vi "Read (I16 Data Ref).vi"(0 "disk streaming in":refnum<class "Disk Streaming.lvclass">, 1 "sample data":refnum<data-value>, 2 "elements in region":u32, 3 "empty elements remaining":u32, 5 "error in (no error)":errorcluster) -> (13 "finished":bool, 14 "disk streaming out":refnum<class "Disk Streaming.lvclass">, 18 "number of pending reads":u32, 19 "error out":errorcluster)   [LabVIEW 2021, in "Disk Streaming.lvclass"]
doc: "Reads data from a file in the streaming process controlled by a disk streaming instance and generates status information. For more information about the disk streaming instance refer to the <B>Open.vi</B> context help.\n\nUse this VI when streaming from disk using the TDMS Advanced Data Reference I/O functions (the disk streaming instance was created by the <B>Open.vi</B> with the <B>disk read (F) / write (T)</B> input set to false and the <B>I/O mode</B> input set to \"Data Reference\"). The streaming process requires the execution of the following sequence in a loop:\n1. Use the <B>Get Next Transfer Size.vi</B> to obtain the number of elements to transfer in the current iteration. If this VI returns zero, then the streaming is complete.\n2. Call the Acquire Write Region FIFO method on the Host to Target FIFO transferring the data to the FPGA Target to acquire the buffer to write with the data read from the file. Use the value returned by the <B>Get Next Transfer Size.vi</B> on the \"Number of Elements\" input of the FIFO method.\n3. Call this VI using the outputs returned by the FIFO method.\n\nInputs:\n\n<B>disk streaming in</B>: Disk streaming instance input.\n\n<B>sample data</B>: External Data Value Reference (EDVR) referencing the array of I16s to write with the data read from the file. Wire the \"Write Region Reference\" output of the FIFO method acquiring the Host to Target FIFO buffer to write to this input.\n\n<B>elements in region</B>: The size of the array of I16s referenced by the EDVR passed on the <B>sample data</B> input. Wire the \"Elements In Region\" output of the FIFO method acquiring the Host to Target FIFO buffer to write to this input.\n\n<B>empty elements remaining</B>: Set this input to the number of additional empty elements remaining in the host DMA buffer that are available for writing. This input is used only in the calculation of the Host DMA buffer utilization status. Wire the \"Empty Elements Remaining\" output of the FIFO method acquiring the Host to Target FIFO buffer to write to this input.\n\nOutputs:\n\n<B>disk streaming out</B>: Disk streaming instance output. Pass this output to the other Disk Streaming VIs to perform the streaming.\n\n<B>number of pending reads</B>: The number of asynchronous reads that are currently running in the background. Use the <B>Get Status.vi</B> to obtain additional status information.\n\n<B>finished</B>: Indicates whether the streaming is finished."
uses:
  Disk Streaming.lvclass
  Disk Streaming.lvclass/Disk Streaming.ctl
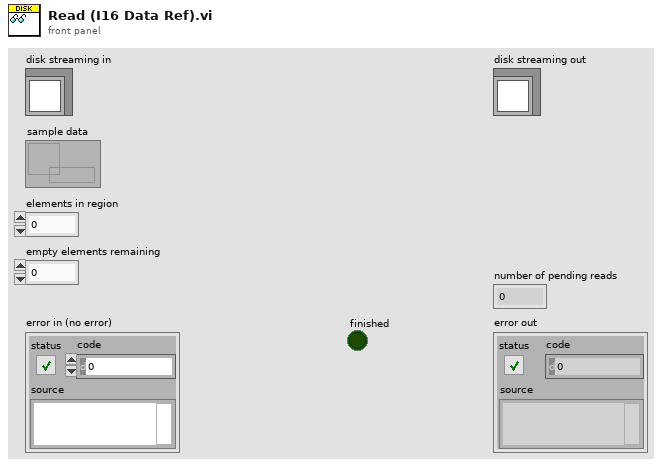
[diagram p1: front panel]
types:
  T1 = typedef "Disk Streaming.lvclass/Data.ctl" = cluster{"tdms file":refnum<k34>, "group name":string, "channel name":string, "max operations":u32, "timeout (s)":dbl, "data type size (bytes)":u64, "writing":bool, "I/O mode":T2, "# of blocks":u32, "block size divisor (bytes)":u32, "file position (elements)":u64, "file size (elements)":i64, "file size (samples)":i64, "block size (elements)":u64, "block size (samples)":u64, "quantum size (elements)":u64, "quantum size (samples)":u64, "samples remaining":i64, "elements transferred":u64, "finished":bool, "preview size":i32, "preview quantum size (elements)":u64, "preview quantum size (samples)":u64, "DMA buffer size (elements)":u32, "pending block sizes (bytes)":u64[]}
  T2 = typedef "Disk Streaming.lvclass/IO mode.ctl" = enum16{"Synchronous", "Asynchronous", "Data Reference"}
  T3 = typedef "Disk Streaming.lvclass/Status.ctl" = cluster{"finished":bool, "Host DMA buffer size (bytes)":u64, "Host DMA buffer utilization (bytes)":u64, "Disk maximum async operations":u32, "Disk pending async operations":u32, "preview data":i16[]}
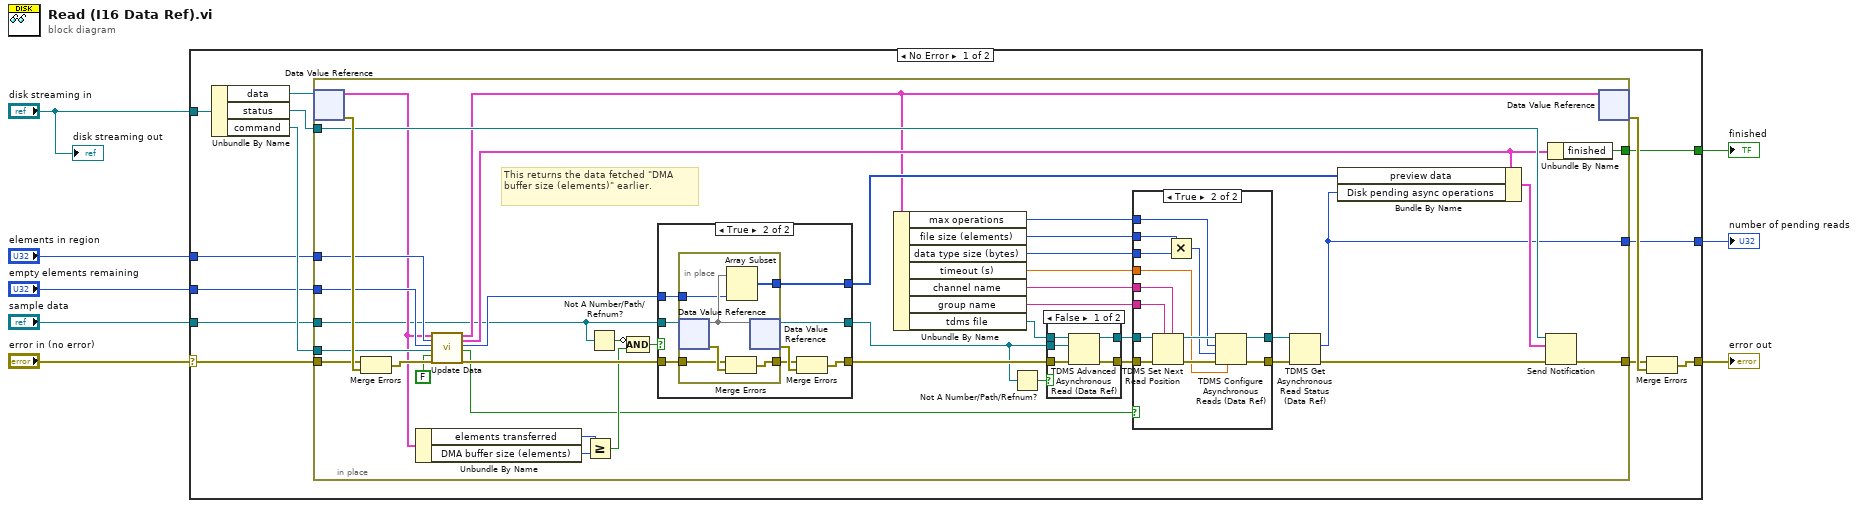
[diagram p0: block diagram]
diagram:
  n1 = case shown="No Error" "error in (no error)" {
    selector: "error in (no error)" -> [w19 w100]
    tunnel: [w18 w100] -> w7
    tunnel: [w16 _] -> w6
    tunnel: "empty elements remaining" -> [w13 _]
    tunnel: "disk streaming in" -> [w15 _]
    tunnel: [w11 _] -> w3
    tunnel: "sample data" -> [w10 _]
    tunnel: "elements in region" -> [w9 _]
    frame No Error {
      n2 = Unbundle By Name(w15) -> ("data"=w14:refnum<data-value>, "status"=w12:refnum<notifier>, "command"=w21:refnum<notifier>)
      n3 = in-place {
        in-place-border: w19 -> [w56]
        in-place-border: [w51] -> w17
        in-place-border: [w35] -> w16
        in-place-border: w21 -> [w53]
        in-place-border: w13 -> [w54]
        in-place-border: w12 -> [w57]
        in-place-border: [w50] -> w11
        in-place-border: w10 -> [w25]
        in-place-border: w9 -> [w44]
        # "This returns the data fetched \"DMA buffer size (elements)\" earlier."
        n4 = in-place-dvr #1(w14) -> (w27:T1, w58:errorcluster)
        n5 = Merge Errors(w56, w58) -> (w59:errorcluster)
        n6 = Unbundle By Name(w27) -> ("elements transferred"=w43:u64, "DMA buffer size (elements)"=w42:u32)
        n7 = call "Update Data.vi"("data in"=w27, "block size (elements)"=w44, "(empty) elements remaining"=w54, "command"=w53, "writing?"=FALSE, "error in (no error)"=w59) -> ("data out"=w26:T1, "status"=w49:T3, "preview size (elements)"=w61:i32, "reopen file"=w24:bool, "error out"=w60:errorcluster)  [unwired: 8 in, 1 out]
        n8 = Greater Or Equal?(x=w43, y=w42) -> (x >= y?=w31:bool)
        n9 = Not A Number/Path/Refnum?(number/path/refnum=w25) -> (NaN/Path/Refnum?=w32:bool)
        n10 = Compound Arithmetic op=AND(invert w32, w31) -> (w30:bool)
        n11 = case shown="True" w30 {
          tunnel: w25 -> [w69 w77]
          tunnel: w60 -> [w70 w76]
          tunnel: w61 -> [_ w75]
          tunnel: [w70 w73] -> w29
          tunnel: [w69 w72] -> w23
          tunnel: [_ w71] -> w28
          frame False {
          }
          frame True {
            n12 = in-place {
              in-place-border: w76 -> [w83]
              in-place-border: [w82] -> w74
              in-place-border: w75 -> [w80]
              in-place-border: [w79] -> w71
              n13 = in-place-dvr #2(w77) -> (w81:i16[], w84:errorcluster)
              n14 = Merge Errors(w83, w84) -> (w82:errorcluster)
              n15 = Array Subset(array=w81, length=w80) -> (w79:i16[])  [unwired: 1 in]
              n16 = in-place-dvr #2(w81) -> (w72:refnum<data-value>, w78:errorcluster)
            }
            n17 = Merge Errors(w74, w78) -> (w73:errorcluster)
          }
        }
        n18 = Unbundle By Name(w26) -> ("max operations"=w33:u32, "file size (elements)"=w34:i64, "data type size (bytes)"=w48:u64, "timeout (s)"=w47:dbl, "channel name"=w46:string, "group name"=w45:string, "tdms file"=w41:refnum<k34>)
        n19 = Not A Number/Path/Refnum?(number/path/refnum=w23) -> (NaN/Path/Refnum?=w22:bool)
        n20 = case shown="False" w22 {
          tunnel: w41 -> [w66 w68]
          tunnel: [w65 w68] -> w40
          tunnel: [w64 w67] -> w39
          tunnel: w29 -> [w63 w67]
          tunnel: w23 -> [w62 _]
          frame False {
            n21 = TDMS Advanced Asynchronous Read (Data Ref)(8:w63, 10:w62, 11:w66) -> (0:w64:errorcluster, 3:w65:refnum<k34>)  [unwired: 1 in, 1 out]
          }
          frame True {
          }
        }
        n22 = case shown="True" w24 {
          tunnel: [w85 w93] -> w37
          tunnel: [w86 w94] -> w38
          tunnel: w40 -> [w86 w97]
          tunnel: w48 -> [_ w90]
          tunnel: w47 -> [_ w91]
          tunnel: w46 -> [_ w99]
          tunnel: w45 -> [_ w98]
          tunnel: w39 -> [w85 w96]
          tunnel: w34 -> [_ w89]
          tunnel: w33 -> [_ w87]
          frame False {
          }
          frame True {
            n23 = TDMS Set Next Read Position(5:w99, 7:w98, 8:w96, 11:w97) -> (0:w92:errorcluster, 3:w95:refnum<k34>)  [unwired: 2 in]
            n24 = Multiply(x=w89, y=w90) -> (x*y=w88:u64)
            n25 = TDMS Configure Asynchronous Reads (Data Ref)(6:w91, 8:w92, 9:w88, 10:w87, 11:w95) -> (0:w93:errorcluster, 3:w94:refnum<k34>)
          }
        }
        n26 = TDMS Get Asynchronous Read Status (Data Ref)(8:w37, 11:w38) -> (0:w36:errorcluster, 2:w35:u32)  [unwired: 1 out]
        n27 = Bundle By Name(cluster=w49, "preview data"=w28, "Disk pending async operations"=w35) -> (w55:T3)
        n28 = Send Notification(notification=w55, notifier=w57, error in (no error)=w36) -> (error out=w51:errorcluster)  [unwired: 1 out]
        n29 = Unbundle By Name(w49) -> ("finished"=w50:bool)
        n30 = in-place-dvr #1(w26) -> (w20:errorcluster)  [unwired: 1 out]
      }
      n31 = Merge Errors(w17, w20) -> (w18:errorcluster)
    }
    frame Error {
    }
  }
  "error out" <- w7
  "number of pending reads" <- w6
  "finished" <- w3
  "disk streaming out" <- "disk streaming in"
